vi "pc_main.vi"() -> ()   [LabVIEW 2013]
panel:
  in  "Acquire On Box 4":bool=TRUE
  in  "Acquire On Box 3":bool=TRUE
  in  "Acquire On Box 2":bool=TRUE
  in  "Acquire On Box 1":bool=TRUE
  in  "Frame Offset":u32=1379862
  in  "Box ID 4":string="M_NA"
  in  "Box ID 3":string="M_NA"
  in  "Box ID 2":string="M_030816_Black6_HFC1"
  in  "Box ID 1":string="M_NA"
  in  "cont_box4":dbl[](array[numeric])
  in  "cont_box3":dbl[](array[numeric])
  in  "cont_box1":dbl[](array[numeric])
  in  "cont_box2":dbl[](array[numeric])
  out "count out 4":i32
  in  "count in 4":i32
  out "count out 3":i32
  in  "count in 3":i32
  in  "count in 1":i32
  out "count out 1":i32
  out "count out 2":i32
  in  "count in 2":i32
  in  "Max Count":i32=1
  in  "Base Path":path=path "Z:/Node1/expt_cooling/data"
  out "Frame Number":u32
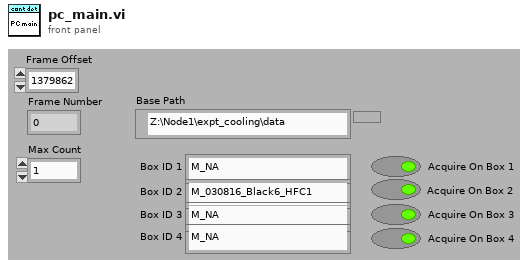
[diagram p1: front panel]
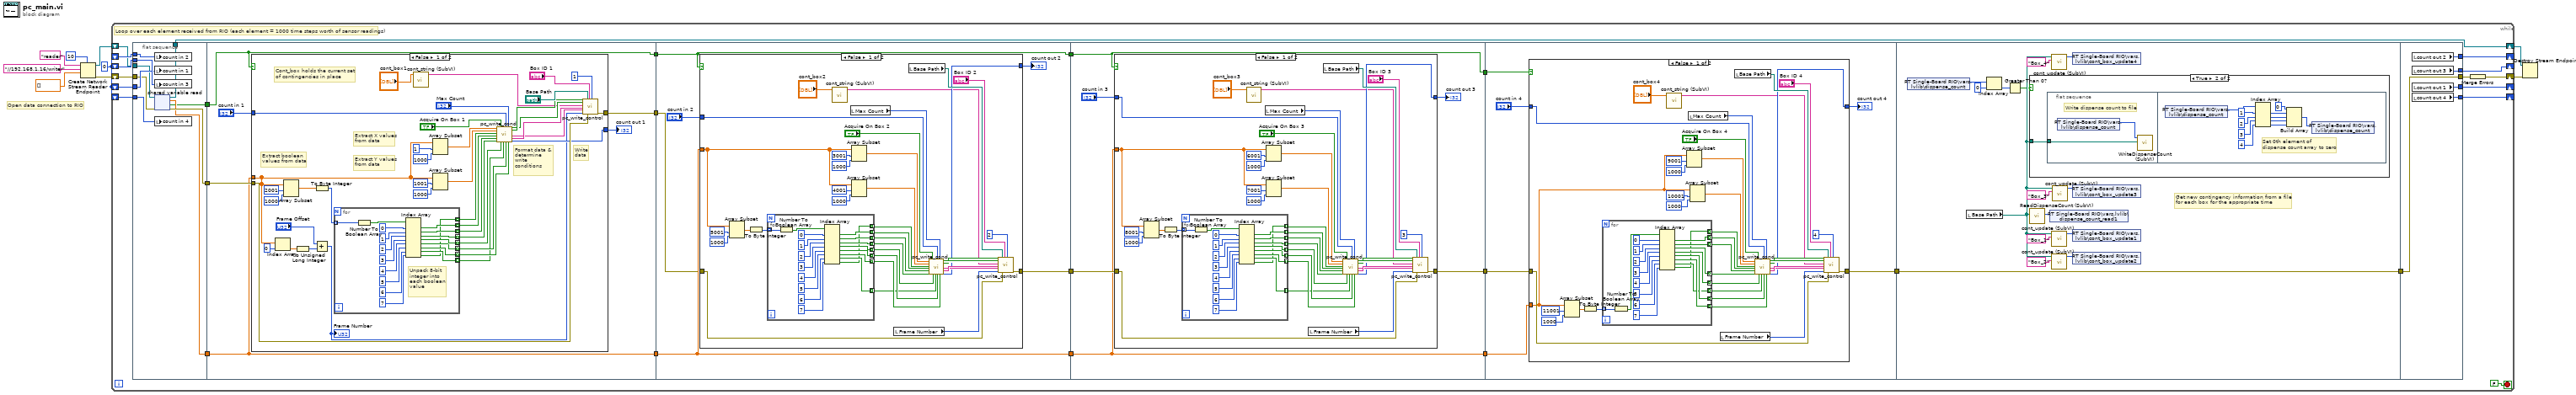
[diagram p0: block diagram]
diagram:
  w1 = 0
  # "Open data connection to RIO"
  n1 = Create Network Stream Reader Endpoint(7:10 ("reader buffer size"), 9:dbl[] [], 10:"//192.168.1.16/writer" ("writer url"), 11:"reader" ("reader name")) -> (0:w2:errorcluster, 3:w5:refnum<k21>)  [unwired: 3 in]
  n2 = while {
    shift-right: [w13] -> w4
    shift-left: w5 -> [w17]
    shift-right: [w36] -> w3
    shift-left: w2 -> [w16]
    shift-right: [w21] -> _
    shift-left: w1 -> [w25]
    shift-right: [w18] -> _
    shift-left: w1 -> [w24]
    shift-right: [w19] -> _
    shift-left: w1 -> [w23]
    shift-right: [w20] -> _
    shift-left: w1 -> [w22]
    stop <- FALSE stop-if-true
    # "Loop over each element received from RIO (each element = 1000 time steps worth of sensor readings)"
    n3 = flat-sequence {
      tunnel: [w41] -> w26
      tunnel: w25 -> [w47]
      tunnel: w24 -> [w46]
      tunnel: w23 -> [w45]
      tunnel: w22 -> [w44]
      tunnel: w17 -> [w43]
      tunnel: w16 -> [w42]
      tunnel: [w40] -> w15
      tunnel: [w39] -> w13
      tunnel: [w38] -> w14
      tunnel: [w50] -> w35
      tunnel: [w49] -> w29
      tunnel: w26 -> [w53]
      tunnel: w15 -> [w50]
      tunnel: w14 -> [w49]
      tunnel: [w48] -> w12
      tunnel: w35 -> [w117]
      tunnel: [w118] -> w33
      tunnel: [w117] -> w32
      tunnel: w29 -> [w114]
      tunnel: [w114] -> w28
      tunnel: w12 -> [w113]
      tunnel: w33 -> [w179]
      tunnel: w32 -> [w175]
      tunnel: [w178] -> w31
      tunnel: [w175] -> w30
      tunnel: w28 -> [w174]
      tunnel: [w174] -> w27
      tunnel: w31 -> [w238]
      tunnel: w30 -> [w236]
      tunnel: w27 -> [w235]
      tunnel: [w237] -> w11
      tunnel: w11 -> [w310]
      tunnel: [w310] -> w10
      tunnel: [w329] -> w34
      tunnel: w10 -> [w329]
      tunnel: [w328] -> w21
      tunnel: [w327] -> w20
      tunnel: [w326] -> w19
      tunnel: [w325] -> w18
      frame #0 {
        n4 = local write "count in 2"(w45) -> ()
        n5 = local write "count in 1"(w44) -> ()
        n6 = local write "count in 3"(w46) -> ()
        n7 = shared-variable-read(w43, w42) -> (w39:refnum<k21>, w41:errorcluster, w38:bool, w40:dbl[])  [unwired: 1 in]
        n8 = local write "count in 4"(w47) -> ()
      }
      frame #1 {
        n9 = case shown="False" w49 {
          tunnel: w50 -> [w65 _]
          tunnel: w53 -> [w83 w112]
          tunnel: [w82 w112] -> w48
          tunnel: "count in 1" -> [w68 w111]
          tunnel: [w67 w111] -> w52
          frame False {
            # "Cont_box holds the current set\nof contingencies in place"
            # "Write\ndata"
            # "Format data &\ndetermine\nwrite \nconditions"
            # "Extract boolean\nvalues from data"
            # "Extract Y values\nfrom data"
            # "Extract X values\nfrom data"
            n10 = Index Array(array=w65, index=0) -> (element=w81:dbl)
            n11 = Array Subset(array=w65, index=2001, length=1000) -> (w86:dbl[])
            n12 = To Unsigned Long Integer(number=w81) -> (unsigned 32bit integer=w60:u32)
            n13 = To Byte Integer(number=w86) -> (8bit integer=w85:i8[])
            n14 = Add(x="Frame Offset", y=w60) -> (x+y=w58:u32)
            "Frame Number" <- w58
            n15 = for {
              tunnel: w85 -> [w110] mode=indexing
              tunnel: [w107] -> w77 mode=indexing
              tunnel: [w102] -> w76 mode=indexing
              tunnel: [w101] -> w75 mode=indexing
              tunnel: [w100] -> w74 mode=indexing
              tunnel: [w99] -> w66 mode=indexing
              tunnel: [w97] -> w57 mode=indexing
              tunnel: [w96] -> w55 mode=indexing
              tunnel: [w93] -> w54 mode=indexing
              # "Unpack 8-bit\ninteger into\neach boolean \nvalue"
              n16 = Number To Boolean Array(number=w110) -> (Boolean array=w109:bool[])
              n17 = Index Array(array=w109, index #1=0 ("index"), index #2=1 ("index"), index #3=2 ("index"), index #4=3 ("index"), index #5=4 ("index"), index #6=5 ("index"), index #7=6 ("index"), index #8=7 ("index")) -> (element #1=w107:bool, element #2=w102:bool, element #3=w101:bool, element #4=w100:bool, element #5=w99:bool, element #6=w97:bool, element #7=w96:bool, element #8=w93:bool)
            }
            n18 = call "cont_string (SubVI).vi"("cont"="cont_box1") -> ("String"=w62:string)  [unwired: 10 in]
            n19 = Array Subset(array=w65, index=1, length=1000) -> (w79:dbl[])
            n20 = Array Subset(array=w65, index=1001, length=1000) -> (w78:dbl[])
            n21 = call "pc_write_cond.vi"("X"=w79, "Y"=w78, "Auto Dispense Flag"=w54, "Touch 1"=w77, "Touch 2"=w76, "Nose Poke"=w75, "Acquire On"="Acquire On Box 1", "Dispense"=w74, "Trial Live"=w55, "Count In"=w68, "Opto On"=w66, "Max Count"="Max Count", "Lick"=w57) -> ("Write Current"=w72:bool, "Write Previous"=w73:bool, "Current Data"=w70:string, "Previous Data"=w71:string, "Count Out"=w67:i32)  [unwired: 2 in]
            n22 = call "pc_write_control.vi"("Write Previous"=w73, "Write Current"=w72, "Cont_info"=w62, "Previous Data"=w71, "Current Data"=w70, "Frame Number"=w58, "Base Path"="Base Path", "error in"=w83, "mouseid"="Box ID 1", "Box Number"=u32 1) -> ("error out"=w82:errorcluster)  [unwired: 9 in]
          }
          frame True {
          }
        }
        "count out 1" <- w52
      }
      frame #2 {
        n23 = case shown="False" w114 {
          tunnel: w117 -> [w127 _]
          tunnel: w113 -> [w145 w173]
          tunnel: [w144 w173] -> w118
          tunnel: "count in 2" -> [w130 w172]
          tunnel: [w129 w172] -> w115
          frame False {
            n24 = Array Subset(array=w127, index=5001, length=1000) -> (w147:dbl[])
            n25 = To Byte Integer(number=w147) -> (8bit integer=w146:i8[])
            n26 = for {
              tunnel: w146 -> [w171] mode=indexing
              tunnel: [w164] -> w139 mode=indexing
              tunnel: [w163] -> w138 mode=indexing
              tunnel: [w162] -> w137 mode=indexing
              tunnel: [w161] -> w136 mode=indexing
              tunnel: [w160] -> w128 mode=indexing
              tunnel: [w158] -> w122 mode=indexing
              tunnel: [w157] -> w120 mode=indexing
              tunnel: [w154] -> w119 mode=indexing
              n27 = Number To Boolean Array(number=w171) -> (Boolean array=w165:bool[])
              n28 = Index Array(array=w165, index #1=0 ("index"), index #2=1 ("index"), index #3=2 ("index"), index #4=3 ("index"), index #5=4 ("index"), index #6=5 ("index"), index #7=6 ("index"), index #8=7 ("index")) -> (element #1=w164:bool, element #2=w163:bool, element #3=w162:bool, element #4=w161:bool, element #5=w160:bool, element #6=w158:bool, element #7=w157:bool, element #8=w154:bool)
            }
            n29 = call "cont_string (SubVI).vi"("cont"="cont_box2") -> ("String"=w124:string)  [unwired: 10 in]
            n30 = local read "Max Count"() -> (w131:i32)
            n31 = Array Subset(array=w127, index=3001, length=1000) -> (w141:dbl[])
            n32 = Array Subset(array=w127, index=4001, length=1000) -> (w140:dbl[])
            n33 = local read "Frame Number"() -> (w142:u32)
            n34 = local read "Base Path"() -> (w143:path)
            n35 = call "pc_write_cond.vi"("X"=w141, "Y"=w140, "Auto Dispense Flag"=w119, "Touch 1"=w139, "Touch 2"=w138, "Nose Poke"=w137, "Acquire On"="Acquire On Box 2", "Dispense"=w136, "Trial Live"=w120, "Count In"=w130, "Opto On"=w128, "Max Count"=w131, "Lick"=w122) -> ("Write Current"=w135:bool, "Write Previous"=w134:bool, "Current Data"=w132:string, "Previous Data"=w133:string, "Count Out"=w129:i32)  [unwired: 2 in]
            n36 = call "pc_write_control.vi"("Write Previous"=w134, "Write Current"=w135, "Cont_info"=w124, "Previous Data"=w133, "Current Data"=w132, "Frame Number"=w142, "Base Path"=w143, "error in"=w145, "mouseid"="Box ID 2", "Box Number"=u32 2) -> ("error out"=w144:errorcluster)  [unwired: 9 in]
          }
          frame True {
          }
        }
        "count out 2" <- w115
      }
      frame #3 {
        n37 = case shown="False" w174 {
          tunnel: w175 -> [w188 _]
          tunnel: w179 -> [w206 w234]
          tunnel: [w205 w234] -> w178
          tunnel: "count in 3" -> [w191 w233]
          tunnel: [w190 w233] -> w176
          frame False {
            n38 = Array Subset(array=w188, index=8001, length=1000) -> (w208:dbl[])
            n39 = To Byte Integer(number=w208) -> (8bit integer=w207:i8[])
            n40 = for {
              tunnel: w207 -> [w232] mode=indexing
              tunnel: [w225] -> w200 mode=indexing
              tunnel: [w224] -> w199 mode=indexing
              tunnel: [w223] -> w198 mode=indexing
              tunnel: [w222] -> w197 mode=indexing
              tunnel: [w221] -> w189 mode=indexing
              tunnel: [w219] -> w183 mode=indexing
              tunnel: [w218] -> w181 mode=indexing
              tunnel: [w215] -> w180 mode=indexing
              n41 = Number To Boolean Array(number=w232) -> (Boolean array=w226:bool[])
              n42 = Index Array(array=w226, index #1=0 ("index"), index #2=1 ("index"), index #3=2 ("index"), index #4=3 ("index"), index #5=4 ("index"), index #6=5 ("index"), index #7=6 ("index"), index #8=7 ("index")) -> (element #1=w225:bool, element #2=w224:bool, element #3=w223:bool, element #4=w222:bool, element #5=w221:bool, element #6=w219:bool, element #7=w218:bool, element #8=w215:bool)
            }
            n43 = call "cont_string (SubVI).vi"("cont"="cont_box3") -> ("String"=w185:string)  [unwired: 10 in]
            n44 = local read "Max Count"() -> (w192:i32)
            n45 = Array Subset(array=w188, index=6001, length=1000) -> (w202:dbl[])
            n46 = Array Subset(array=w188, index=7001, length=1000) -> (w201:dbl[])
            n47 = local read "Frame Number"() -> (w203:u32)
            n48 = local read "Base Path"() -> (w204:path)
            n49 = call "pc_write_cond.vi"("X"=w202, "Y"=w201, "Auto Dispense Flag"=w180, "Touch 1"=w200, "Touch 2"=w199, "Nose Poke"=w198, "Acquire On"="Acquire On Box 3", "Dispense"=w197, "Trial Live"=w181, "Count In"=w191, "Opto On"=w189, "Max Count"=w192, "Lick"=w183) -> ("Write Current"=w196:bool, "Write Previous"=w195:bool, "Current Data"=w193:string, "Previous Data"=w194:string, "Count Out"=w190:i32)  [unwired: 2 in]
            n50 = call "pc_write_control.vi"("Write Previous"=w195, "Write Current"=w196, "Cont_info"=w185, "Previous Data"=w194, "Current Data"=w193, "Frame Number"=w203, "Base Path"=w204, "error in"=w206, "mouseid"="Box ID 3", "Box Number"=u32 3) -> ("error out"=w205:errorcluster)  [unwired: 9 in]
          }
          frame True {
          }
        }
        "count out 3" <- w176
      }
      frame #4 {
        n51 = case shown="False" w235 {
          tunnel: w236 -> [w249 _]
          tunnel: w238 -> [w267 w295]
          tunnel: [w266 w295] -> w237
          tunnel: "count in 4" -> [w252 w294]
          tunnel: [w251 w294] -> w239
          frame False {
            n52 = Array Subset(array=w249, index=11001, length=1000) -> (w269:dbl[])
            n53 = To Byte Integer(number=w269) -> (8bit integer=w268:i8[])
            n54 = for {
              tunnel: w268 -> [w293] mode=indexing
              tunnel: [w286] -> w261 mode=indexing
              tunnel: [w285] -> w260 mode=indexing
              tunnel: [w284] -> w259 mode=indexing
              tunnel: [w283] -> w258 mode=indexing
              tunnel: [w282] -> w250 mode=indexing
              tunnel: [w280] -> w244 mode=indexing
              tunnel: [w279] -> w242 mode=indexing
              tunnel: [w276] -> w241 mode=indexing
              n55 = Number To Boolean Array(number=w293) -> (Boolean array=w287:bool[])
              n56 = Index Array(array=w287, index #1=0 ("index"), index #2=1 ("index"), index #3=2 ("index"), index #4=3 ("index"), index #5=4 ("index"), index #6=5 ("index"), index #7=6 ("index"), index #8=7 ("index")) -> (element #1=w286:bool, element #2=w285:bool, element #3=w284:bool, element #4=w283:bool, element #5=w282:bool, element #6=w280:bool, element #7=w279:bool, element #8=w276:bool)
            }
            n57 = call "cont_string (SubVI).vi"("cont"="cont_box4") -> ("String"=w246:string)  [unwired: 10 in]
            n58 = Array Subset(array=w249, index=9001, length=1000) -> (w263:dbl[])
            n59 = local read "Max Count"() -> (w253:i32)
            n60 = Array Subset(array=w249, index=10001, length=1000) -> (w262:dbl[])
            n61 = local read "Frame Number"() -> (w264:u32)
            n62 = local read "Base Path"() -> (w265:path)
            n63 = call "pc_write_cond.vi"("X"=w263, "Y"=w262, "Auto Dispense Flag"=w241, "Touch 1"=w261, "Touch 2"=w260, "Nose Poke"=w259, "Acquire On"="Acquire On Box 4", "Dispense"=w258, "Trial Live"=w242, "Count In"=w252, "Opto On"=w250, "Max Count"=w253, "Lick"=w244) -> ("Write Current"=w257:bool, "Write Previous"=w256:bool, "Current Data"=w254:string, "Previous Data"=w255:string, "Count Out"=w251:i32)  [unwired: 2 in]
            n64 = call "pc_write_control.vi"("Write Previous"=w256, "Write Current"=w257, "Cont_info"=w246, "Previous Data"=w255, "Current Data"=w254, "Frame Number"=w264, "Base Path"=w265, "error in"=w267, "mouseid"="Box ID 4", "Box Number"=u32 4) -> ("error out"=w266:errorcluster)  [unwired: 9 in]
          }
          frame True {
          }
        }
        "count out 4" <- w239
      }
      frame #5 {
        # "Get new contingency information from a file\nfor each box for the appropriate time"
        n65 = shared-variable "RT Single-Board RIO\\vars.lvlib\\dispense_count"() -> (w301:u16[])  [unwired: 1 in, 1 out]
        n66 = local read "Base Path"() -> (w299:path)
        n67 = Index Array(array=w301, index=0) -> (element=w296:u16)
        n68 = Greater Than 0?(x=w296) -> (x > 0?=w297:bool)
        n69 = case shown="True" w297 {
          tunnel: w299 -> [_ w311]
          frame False {
          }
          frame True {
            n70 = flat-sequence {
              tunnel: w311 -> [w313]
              frame #0 {
                # "Write dispense count to file"
                n71 = shared-variable "RT Single-Board RIO\\vars.lvlib\\dispense_count"() -> (w312:u16[])  [unwired: 1 in, 1 out]
                n72 = call "WriteDispenseCount (SubVI).vi"("Base Path"=w313, "Array of UInt16"=w312) -> ()  [unwired: 10 in]
              }
              frame #1 {
                # "Set 0th element of\ndispense count array to zero"
                n73 = shared-variable "RT Single-Board RIO\\vars.lvlib\\dispense_count"() -> (w324:u16[])  [unwired: 1 in, 1 out]
                n74 = Index Array(array=w324, index #1=1 ("index"), index #2=2 ("index"), index #3=3 ("index"), index #4=4 ("index")) -> (element #1=w321:u16, element #2=w320:u16, element #3=w319:u16, element #4=w318:u16)
                n75 = Build Array(u16 0 ("element"), w321, w320, w319, w318) -> (w322:u16[])
                n76 = shared-variable "RT Single-Board RIO\\vars.lvlib\\dispense_count"(w322) -> ()  [unwired: 1 in, 1 out]
              }
            }
          }
        }
        n77 = call "ReadDispenseCount (SubVI).vi"("Base Path"=w299) -> ("appended array"=w298:i32[])  [unwired: 10 in]
        n78 = shared-variable "RT Single-Board RIO\\vars.lvlib\\dispense_count_read1"(w298) -> ()  [unwired: 1 in, 1 out]
        n79 = call "cont_update (SubVI).vi"("name or relative path"="Box_4", "Base Path"=w299) -> ("Array Out"=w302:i32[])  [unwired: 9 in]
        n80 = call "cont_update (SubVI).vi"("name or relative path"="Box_1", "Base Path"=w299) -> ("Array Out"=w308:i32[])  [unwired: 9 in]
        n81 = call "cont_update (SubVI).vi"("name or relative path"="Box_2", "Base Path"=w299) -> ("Array Out"=w304:i32[])  [unwired: 9 in]
        n82 = call "cont_update (SubVI).vi"("name or relative path"="Box_3", "Base Path"=w299) -> ("Array Out"=w303:i32[])  [unwired: 9 in]
        n83 = shared-variable "RT Single-Board RIO\\vars.lvlib\\cont_box_update4"(w302) -> ()  [unwired: 1 in, 1 out]
        n84 = shared-variable "RT Single-Board RIO\\vars.lvlib\\cont_box_update3"(w303) -> ()  [unwired: 1 in, 1 out]
        n85 = shared-variable "RT Single-Board RIO\\vars.lvlib\\cont_box_update1"(w308) -> ()  [unwired: 1 in, 1 out]
        n86 = shared-variable "RT Single-Board RIO\\vars.lvlib\\cont_box_update2"(w304) -> ()  [unwired: 1 in, 1 out]
      }
      frame #6 {
        n87 = local read "count out 2"() -> (w326:i32)
        n88 = local read "count out 3"() -> (w325:i32)
        n89 = local read "count out 1"() -> (w327:i32)
        n90 = local read "count out 4"() -> (w328:i32)
      }
    }
    n91 = Merge Errors(w34) -> (w36:errorcluster)
  }
  n92 = Destroy Stream Endpoint(8:w3, 11:w4) -> ()  [unwired: 1 out]
